vi "Build Do.vi"(6 "Wiring Spec":T1, 8 "error in (no error)":errorcluster, 10 "Do VI":refnum<vi>, 11 "CS++Actor in":refnum<class "CS++Actor.lvclass">) -> (0 "error out":errorcluster, 3 "CS++Actor out":refnum<class "CS++Actor.lvclass">)   [LabVIEW 2014, in "CS++Actor.lvlib" / "CS++Actor.lvclass"]
doc: "Creates the Do.vi for the new message."
uses:
  CS++Actor.lvclass
  CS++Actor.lvclass/CS++Actor.ctl
  <vilib>/Utility/traverseref.llb/TRef TravTarget.ctl
  <vilib>/Utility/traverseref.llb/VI Scripting - Traverse.lvlib
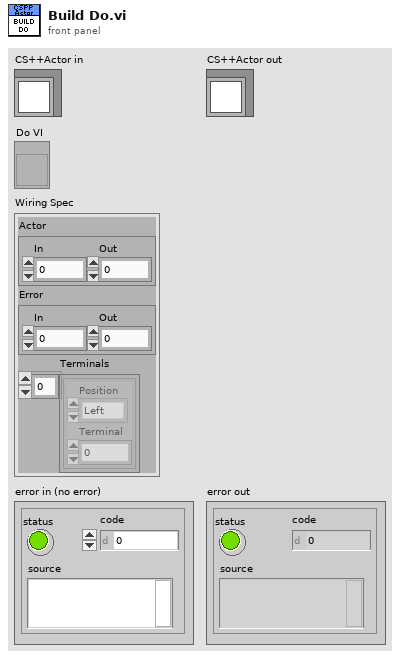
[diagram p1: front panel]
types:
  T1 = cluster{"Actor":cluster{"In":i32, "Out":i32}, "Error":cluster{"In":i32, "Out":i32}, "Terminals":cluster{"Position":enum16{"Left", "Top", "Bottom", "Right"}, "Terminal":i32}[]}
  T2 = enum16{"Replace Class Controls/Constants", "Prepare SubVI", "Wire Method Inputs"}
  T3 = typedef "TRef TravTarget.ctl" = enum16{"FP", "BD", "Other"}
  T4 = cluster{"Position":enum16{"Left", "Top", "Bottom", "Right"}, "Terminal":i32}[]
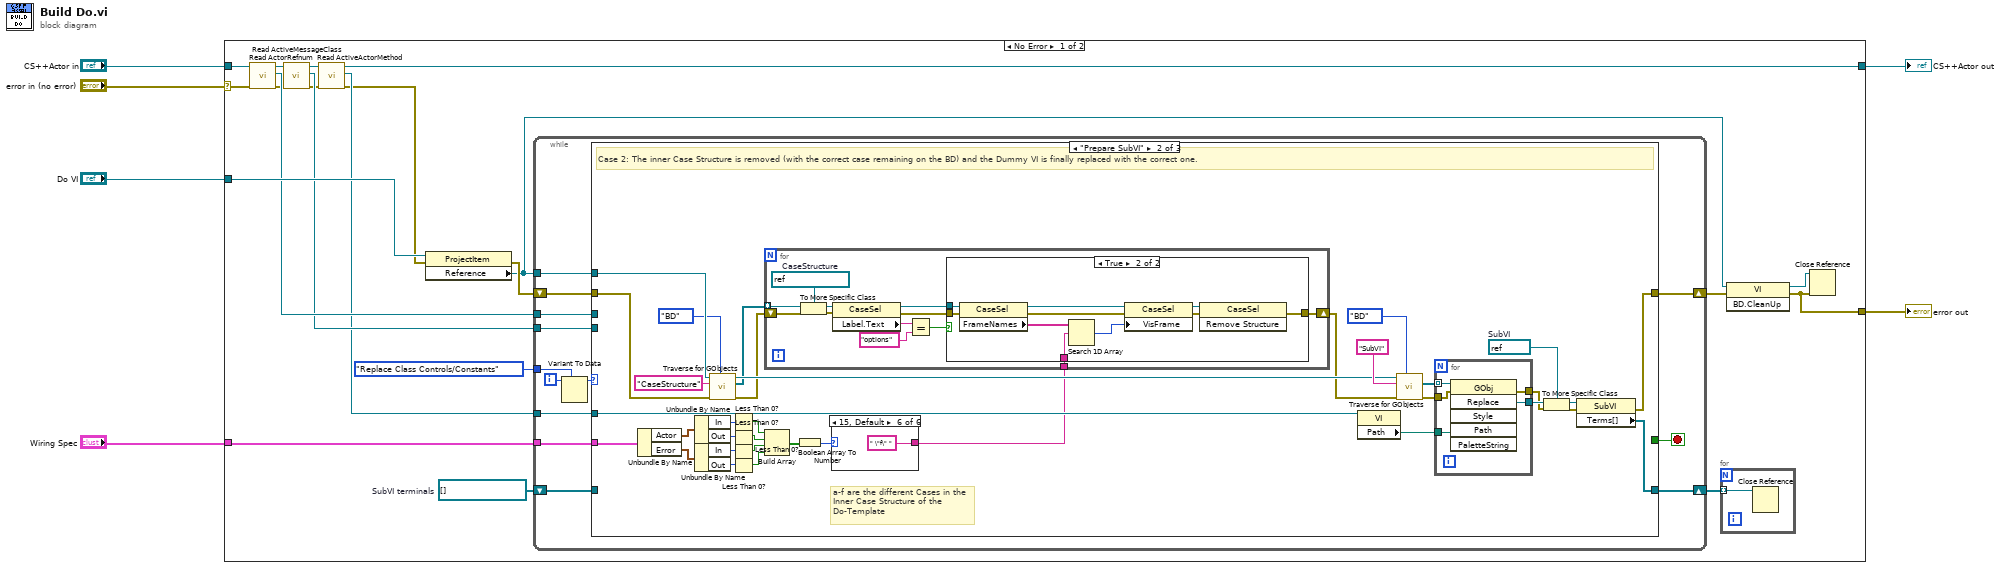
[diagram p0: block diagram]
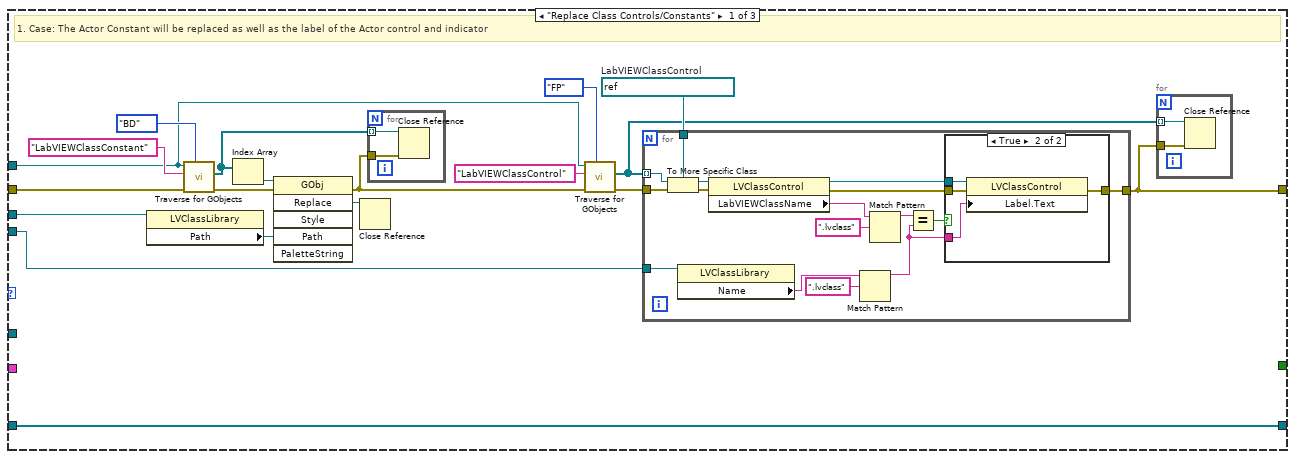
[diagram p2: hidden frame]
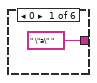
[diagram p5: hidden frame]
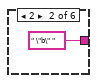
[diagram p6: hidden frame]
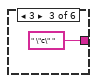
[diagram p7: hidden frame]
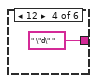
[diagram p8: hidden frame]
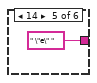
[diagram p9: hidden frame]
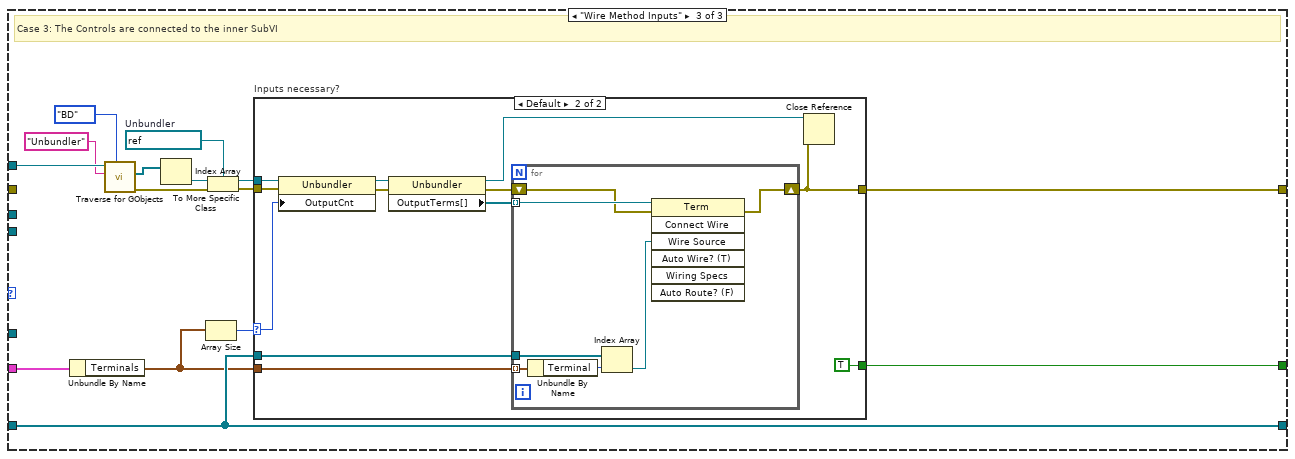
[diagram p10: hidden frame]
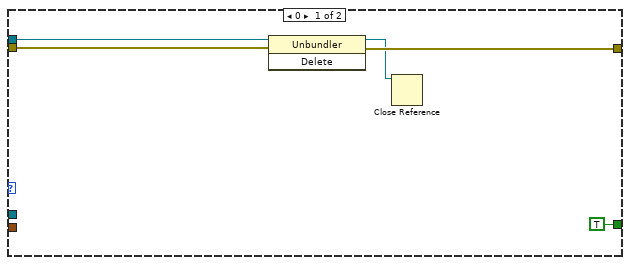
[diagram p11: hidden frame]
diagram:
  n1 = case shown="No Error" "error in (no error)" {
    selector: "error in (no error)" -> [w7 w194]
    tunnel: "Do VI" -> [w27 _]
    tunnel: "Wiring Spec" -> [w25 _]
    tunnel: [w18 w194] -> w4
    tunnel: "CS++Actor in" -> [w17 w195]
    tunnel: [w8 w195] -> w2
    frame No Error {
      w21 = refnum<vi>[] []  # SubVI terminals
      n2 = call "Read ActorRefnum.vi"("error in (no error)"=w7, "CS++Actor in"=w17) -> ("error out"=w14:errorcluster, "ActorRefnum"=w16:refnum<vi>, "CS++Actor out"=w15:refnum<class "CS++Actor.lvclass">)  [unwired: 7 in]
      n3 = call "Read ActiveMessageClass.vi"("error in (no error)"=w14, "CS++Actor in"=w15) -> ("error out"=w11:errorcluster, "ActiveMessageClass"=w13:refnum<vi>, "CS++Actor out"=w12:refnum<class "CS++Actor.lvclass">)  [unwired: 7 in]
      n4 = call "Read ActiveActorMethod.vi"("error in (no error)"=w11, "CS++Actor in"=w12) -> ("error out"=w9:errorcluster, "ActiveActorMethod"=w10:refnum<vi>, "CS++Actor out"=w8:refnum<class "CS++Actor.lvclass">)  [unwired: 7 in]
      n5 = property class="ProjectItem"(reference=w27, error in=w9) -> (error out=w26:errorcluster, "Reference"=w19:refnum<vi>)  [unwired: 1 out]
      n6 = while {
        tunnel: w19 -> [w41]
        tunnel: w25 -> [w39]
        shift-right: [w38] -> w24
        shift-left: w26 -> [w40]
        tunnel: T2."Replace Class Controls/Constants" -> [w36]
        tunnel: w16 -> [w34]
        tunnel: w10 -> [w33]
        shift-right: [w31] -> w20
        shift-left: w21 -> [w30]
        tunnel: w13 -> [w29]
        i -> [w37]
        stop <- w32 stop-if-true
        n7 = Variant To Data(type=w36, Variant=w37) -> (data=w35:T2)  [unwired: 1 in, 1 out]
        n8 = case shown="\"Prepare SubVI\"" w35 {
          tunnel: w41 -> [w49 w120 w169]
          tunnel: w40 -> [w54 w119 _]
          tunnel: w39 -> [_ w118 w162]
          tunnel: [w42 w86 w158] -> w38
          tunnel: w34 -> [w55 _ _]
          tunnel: w33 -> [_ w117 _]
          tunnel: [_ _ w155] -> w32
          tunnel: [w51 w116 w157] -> w31
          tunnel: w30 -> [w51 _ w157]
          tunnel: w29 -> [w44 _ _]
          frame "Replace Class Controls/Constants" {
            w47 = refnum<vi> refnum  # LabVIEWClassControl
            # "1. Case: The Actor Constant will be replaced as well as the label of the Actor control and indicator"
            n9 = property class="LVClassLibrary"(reference=w55) -> ("Path"=w58:path)  [unwired: 1 in, 2 out]
            n10 = call <vilib>:"Traverse for GObjects.vi"("Traverse Target"=TRef_TravTarget."BD", "error in (no error)"=w54, "Class Name"="LabVIEWClassConstant", "VI Refnum"=w49) -> ("error out"=w59:errorcluster, "References"=w53:refnum<vi>[])  [unwired: 4 in, 2 out]
            n11 = Index Array(array=w53) -> (element=w57:refnum<vi>)  [unwired: 1 in]
            n12 = invoke class="GObj" method="Replace"(reference=w57, error in=w59, "Path"=w58) -> (error out=w50:errorcluster, "Replace"=w52:refnum<vi>)  [unwired: 3 in, 4 out]
            n13 = Close Reference(reference=w52) -> ()  [unwired: 1 in, 1 out]
            n14 = for {
              tunnel: w53 -> [w64] mode=indexing
              tunnel: w50 -> [w63]
              n15 = Close Reference(reference=w64, error in (no error)=w63) -> ()  [unwired: 1 out]
            }
            n16 = call <vilib>:"Traverse for GObjects.vi"("Traverse Target"=TRef_TravTarget."FP", "error in (no error)"=w50, "Class Name"="LabVIEWClassControl", "VI Refnum"=w49) -> ("error out"=w45:errorcluster, "References"=w43:refnum<vi>[])  [unwired: 4 in, 2 out]
            n17 = for {
              tunnel: w47 -> [w80]
              tunnel: w45 -> [w79]
              tunnel: w43 -> [w78] mode=indexing
              tunnel: w44 -> [w73]
              tunnel: [w75] -> w42
              n18 = To More Specific Class(target class=w80, reference=w78, error in=w79) -> (specific class reference=w74:refnum<vi>, error out=w76:errorcluster)
              n19 = property class="LVClassLibrary"(reference=w73) -> ("Name"=w71:string)  [unwired: 1 in, 2 out]
              n20 = property class="LVClassControl"(reference=w74, error in=w76) -> (reference out=w77:refnum<vi>, error out=w65:errorcluster, "LabVIEWClassName"=w67:string)
              n21 = Match Pattern(string=w71, regular expression=".lvclass") -> (before substring=w70:string)  [unwired: 1 in, 3 out]
              n22 = Match Pattern(string=w67, regular expression=".lvclass") -> (before substring=w66:string)  [unwired: 1 in, 3 out]
              n23 = Equal?(x=w66, y=w70) -> (x = y?=w72:bool)
              n24 = case shown="True" w72 {
                tunnel: w77 -> [_ w85]
                tunnel: [w81 w82] -> w75
                tunnel: w70 -> [_ w84]
                tunnel: w65 -> [w81 w83]
                frame False {
                }
                frame True {
                  n25 = property class="LVClassControl"(reference=w85, error in=w83, "Label.Text"=w84) -> (error out=w82:errorcluster)  [unwired: 1 out]
                }
              }
            }
            n26 = for {
              tunnel: w43 -> [w62] mode=indexing
              tunnel: w42 -> [w61]
              n27 = Close Reference(reference=w62, error in (no error)=w61) -> ()  [unwired: 1 out]
            }
          }
          frame "Prepare SubVI" {
            w89 = refnum<vi> refnum  # SubVI
            # "a-f are the different Cases in the\nInner Case Structure of the \nDo-Template"
            # "Case 2: The inner Case Structure is removed (with the correct case remaining on the BD) and the Dummy VI is finally replaced with the correct one."
            n28 = Unbundle By Name(w118) -> ("Actor"=w111:cluster{"In":i32, "Out":i32}, "Error"=w110:cluster{"In":i32, "Out":i32})
            n29 = Unbundle By Name(w111) -> ("In"=w109:i32, "Out"=w108:i32)
            n30 = Unbundle By Name(w110) -> ("In"=w107:i32, "Out"=w106:i32)
            n31 = call <vilib>:"Traverse for GObjects.vi"("Traverse Target"=TRef_TravTarget."BD", "error in (no error)"=w119, "Class Name"="CaseStructure", "VI Refnum"=w120) -> ("error out"=w94:errorcluster, "References"=w96:refnum<vi>[], "dup VI Refnum"=w99:refnum<vi>)  [unwired: 4 in, 1 out]
            n32 = Less Than 0?(x=w109) -> (x < 0?=w105:bool)
            n33 = Less Than 0?(x=w108) -> (x < 0?=w104:bool)
            n34 = Less Than 0?(x=w107) -> (x < 0?=w103:bool)
            n35 = Less Than 0?(x=w106) -> (x < 0?=w102:bool)
            n36 = Build Array(w105, w104, w103, w102) -> (w101:bool[])
            n37 = Boolean Array To Number(Boolean array=w101) -> (number=w100:u32)
            n38 = case shown="15, Default" w100 {
              tunnel: [" \"a\" " " \"b\" " " \"c\" " " \"d\" " " \"e\" " " \"f\" "] -> w95
              frame 0 {
              }
              frame 2 {
              }
              frame 3 {
              }
              frame 12 {
              }
              frame 14 {
              }
              frame 15, Default {
              }
            }
            n39 = for {
              tunnel: w96 -> [w132] mode=indexing
              tunnel: w95 -> [w123]
              shift-right: [w121] -> w93
              shift-left: w94 -> [w122]
              w131 = refnum<vi> refnum  # CaseStructure
              n40 = To More Specific Class(target class=w131, reference=w132, error in=w122) -> (specific class reference=w130:refnum<vi>, error out=w129:errorcluster)
              n41 = property class="CaseSel"(reference=w130, error in=w129) -> (reference out=w125:refnum<vi>, error out=w124:errorcluster, "Label.Text"=w128:string)
              n42 = Equal?(x=w128, y="options") -> (x = y?=w126:bool)
              n43 = case shown="True" w126 {
                tunnel: w125 -> [_ w141]
                tunnel: w124 -> [w133 w139]
                tunnel: w123 -> [_ w135]
                tunnel: [w133 w134] -> w121
                frame False {
                }
                frame True {
                  n44 = property class="CaseSel"(reference=w141, error in=w139) -> (reference out=w140:refnum<vi>, error out=w138:errorcluster, "FrameNames"=w137:string[])
                  n45 = Search 1D Array(1D array=w137, element=w135) -> (index of element=w136:i32)  [unwired: 1 in]
                  n46 = property class="CaseSel"(reference=w140, error in=w138, "VisFrame"=w136) -> (reference out=w143:refnum<vi>, error out=w142:errorcluster)
                  n47 = invoke class="CaseSel" method="Remove Structure"(reference=w143, error in=w142) -> (error out=w134:errorcluster)  [unwired: 1 in, 2 out]
                }
              }
            }
            n48 = property class="VI"(reference=w117) -> ("Path"=w112:path)  [unwired: 1 in, 2 out]
            n49 = call <vilib>:"Traverse for GObjects.vi"("Traverse Target"=TRef_TravTarget."BD", "error in (no error)"=w93, "Class Name"="SubVI", "VI Refnum"=w99) -> ("error out"=w88:errorcluster, "References"=w113:refnum<vi>[])  [unwired: 4 in, 2 out]
            n50 = for {
              tunnel: w113 -> [w154] mode=indexing
              tunnel: w112 -> [w153]
              tunnel: [w152] -> w91
              tunnel: w88 -> [w151]
              tunnel: [w150] -> w87
              n51 = invoke class="GObj" method="Replace"(reference=w154, error in=w151, "Path"=w153) -> (error out=w150:errorcluster, "Replace"=w152:refnum<vi>)  [unwired: 3 in, 4 out]
            }
            n52 = To More Specific Class(target class=w89, reference=w91, error in=w87) -> (specific class reference=w92:refnum<vi>, error out=w90:errorcluster)
            n53 = property class="SubVI"(reference=w92, error in=w90) -> (error out=w86:errorcluster, "Terms[]"=w116:refnum<vi>[])  [unwired: 1 out]
          }
          frame "Wire Method Inputs" {
            w163 = refnum<vi> refnum  # Unbundler
            # "Case 3: The Controls are connected to the inner SubVI"
            n54 = Unbundle By Name(w162) -> ("Terminals"=w156:T4)
            n55 = call <vilib>:"Traverse for GObjects.vi"("Traverse Target"=TRef_TravTarget."BD", "Class Name"="Unbundler", "VI Refnum"=w169) -> ("error out"=w164:errorcluster, "References"=w166:refnum<vi>[])  [unwired: 5 in, 2 out]
            n56 = Index Array(array=w166) -> (element=w165:refnum<vi>)  [unwired: 1 in]
            n57 = Array Size(array=w156) -> (size(s)=w161:i32)
            n58 = To More Specific Class(target class=w163, reference=w165, error in=w164) -> (specific class reference=w160:refnum<vi>, error out=w159:errorcluster)
            n59 = case "Inputs necessary?" shown="Default" w161 {
              selector: w161 -> [_ w181]
              tunnel: w160 -> [w174 w179]
              tunnel: w157 -> [_ w184]
              tunnel: w159 -> [w173 w176]
              tunnel: [w172 w177] -> w158
              tunnel: w156 -> [_ w186]
              tunnel: [TRUE TRUE] -> w155
              frame 0 {
                n60 = invoke class="Unbundler" method="Delete"(reference=w174, error in=w173) -> (reference out=w171:refnum<vi>, error out=w172:errorcluster)  [unwired: 1 in, 1 out]
                n61 = Close Reference(reference=w171) -> ()  [unwired: 1 in, 1 out]
              }
              frame Default {
                n62 = property class="Unbundler"(reference=w179, error in=w176, "OutputCnt"=w181) -> (reference out=w182:refnum<vi>, error out=w180:errorcluster)
                n63 = property class="Unbundler"(reference=w182, error in=w180) -> (reference out=w178:refnum<vi>, error out=w183:errorcluster, "OutputTerms[]"=w185:refnum<vi>[])
                n64 = for {
                  tunnel: w186 -> [w188] mode=indexing
                  tunnel: w185 -> [w193] mode=indexing
                  tunnel: w184 -> [w192]
                  shift-right: [w189] -> w177
                  shift-left: w183 -> [w190]
                  n65 = Unbundle By Name(w188) -> ("Terminal"=w187:i32)
                  n66 = Index Array(array=w192, index=w187) -> (element=w191:refnum<vi>)
                  n67 = invoke class="Term" method="Connect Wire"(reference=w193, error in=w190, "Wire Source"=w191) -> (error out=w189:errorcluster)  [unwired: 4 in, 6 out]
                }
                n68 = Close Reference(reference=w178, error in (no error)=w177) -> ()  [unwired: 1 out]
              }
            }
          }
        }
      }
      n69 = for {
        tunnel: w20 -> [w28] mode=indexing
        n70 = Close Reference(reference=w28) -> ()  [unwired: 1 in, 1 out]
      }
      n71 = invoke class="VI" method="BD.CleanUp"(reference=w19, error in=w24) -> (reference out=w23:refnum<vi>, error out=w18:errorcluster)  [unwired: 1 in, 1 out]
      n72 = Close Reference(reference=w23, error in (no error)=w18) -> ()  [unwired: 1 out]
    }
    frame Error {
    }
  }
  "error out" <- w4
  "CS++Actor out" <- w2
